vi "Get Gamepads.vi"() -> (1 "Secondary":T1, 2 "Driver":T1)   [LabVIEW 2011]
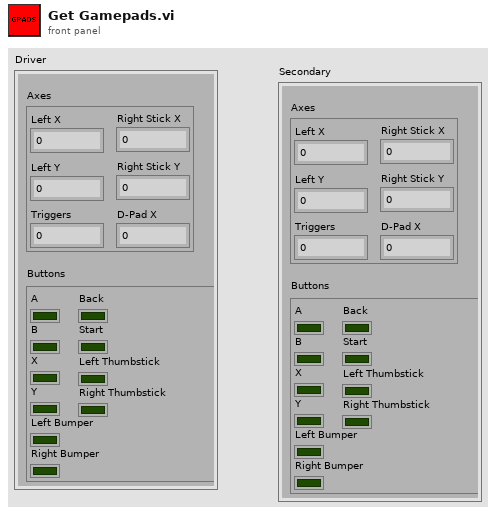
[diagram p1: front panel]
types:
  T1 = cluster{"Buttons":cluster{"A":bool, "B":bool, "X":bool, "Y":bool, "Left Bumper":bool, "Right Bumper":bool, "Back":bool, "Start":bool, "Left Thumbstick":bool, "Right Thumbstick":bool}, "Axes":cluster{"Left X ":dbl, "Left Y":dbl, "Triggers":dbl, "Right Stick X":dbl, "Right Stick Y":dbl, "D-Pad X":dbl}}
  T2 = typedef "WPI_JoystickButtonState.ctl" = cluster{"Button 1":bool, "Button 2":bool, "Button 3":bool, "Button 4":bool, "Button 5":bool, "Button 6":bool, "Button 7":bool, "Button 8":bool, "Button 9":bool, "Button 10":bool, "Button 11":bool, "Button 12":bool}
  T3 = cluster{"Buttons":T2, "Axes":cluster{"axis 1 (x)":dbl, "axis 2 (y)":dbl, "axis 3 (throttle)":dbl, "axis 4":dbl, "axis 5":dbl, "axis 6":dbl}}
  T4 = cluster{"axis 1 (x)":dbl, "axis 2 (y)":dbl, "axis 3 (throttle)":dbl, "axis 4":dbl, "axis 5":dbl, "axis 6":dbl}
  T5 = cluster{"A":bool, "B":bool, "X":bool, "Y":bool, "Left Bumper":bool, "Right Bumper":bool, "Back":bool, "Start":bool, "Left Thumbstick":bool, "Right Thumbstick":bool}
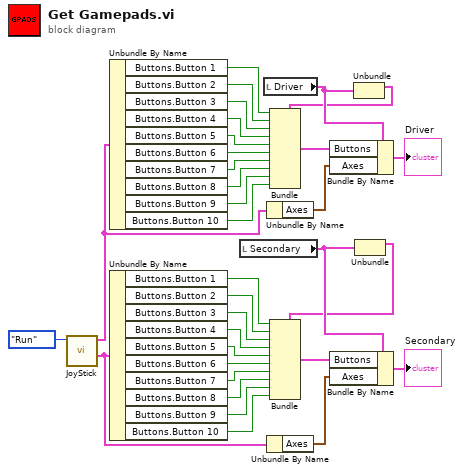
[diagram p0: block diagram]
diagram:
  n1 = call "JoyStick.vi"("Enum"=enum16{"Init", "Run", "End"}."Run") -> ("JoyStick 3"=w32:T3, "JoyStick 1"=w9:T3)  [unwired: 7 in, 2 out]
  n2 = Unbundle By Name(w9) -> ("Buttons.Button 1"=w10:bool, "Buttons.Button 2"=w11:bool, "Buttons.Button 3"=w12:bool, "Buttons.Button 4"=w13:bool, "Buttons.Button 5"=w14:bool, "Buttons.Button 6"=w15:bool, "Buttons.Button 7"=w16:bool, "Buttons.Button 8"=w17:bool, "Buttons.Button 9"=w18:bool, "Buttons.Button 10"=w6:bool)
  n3 = Unbundle By Name(w32) -> ("Buttons.Button 1"=w28:bool, "Buttons.Button 2"=w27:bool, "Buttons.Button 3"=w26:bool, "Buttons.Button 4"=w25:bool, "Buttons.Button 5"=w24:bool, "Buttons.Button 6"=w23:bool, "Buttons.Button 7"=w22:bool, "Buttons.Button 8"=w21:bool, "Buttons.Button 9"=w20:bool, "Buttons.Button 10"=w19:bool)
  n4 = local read "Secondary"() -> (w2:T1)
  n5 = local read "Driver"() -> (w4:T1)
  n6 = Unbundle By Name(w9) -> ("Axes"=w5:T4)
  n7 = Unbundle By Name(w32) -> ("Axes"=w29:T4)
  n8 = Unbundle(w4) -> ("Buttons"=w3:T5)  [unwired: 1 out]
  n9 = Bundle(cluster=w3, "A"=w10, "B"=w11, "X"=w12, "Y"=w13, "Left Bumper"=w14, "Right Bumper"=w15, "Back"=w16, "Start"=w17, "Left Thumbstick"=w18, "Right Thumbstick"=w6) -> (w8:T5)
  n10 = Bundle By Name(cluster=w4, "Buttons"=w8, "Axes"=w5) -> (→"Driver":T1)
  n11 = Unbundle(w2) -> ("Buttons"=w1:T5)  [unwired: 1 out]
  n12 = Bundle(cluster=w1, "A"=w28, "B"=w27, "X"=w26, "Y"=w25, "Left Bumper"=w24, "Right Bumper"=w23, "Back"=w22, "Start"=w21, "Left Thumbstick"=w20, "Right Thumbstick"=w19) -> (w7:T5)
  n13 = Bundle By Name(cluster=w2, "Buttons"=w7, "Axes"=w29) -> (→"Secondary":T1)
